vi "Full Stock venta.vi"(7 "Inventario/ventas":bool=TRUE, 8 "error in (no error)":errorcluster, 10 "Ubicacion":string, 11 "Full pedido":string[][](array[string])) -> (0 "error out":errorcluster, 3 "Sobrantes":string[][](array[string]))   [LabVIEW 2018]
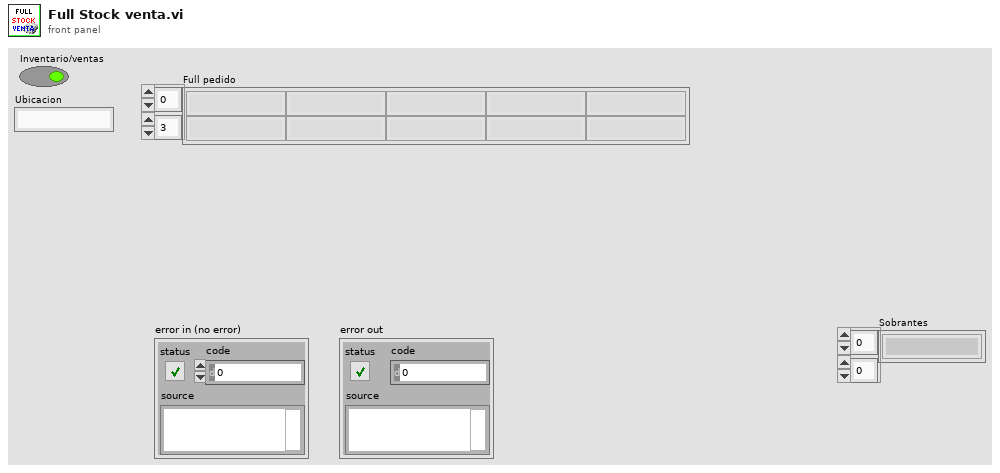
[diagram p1: front panel]
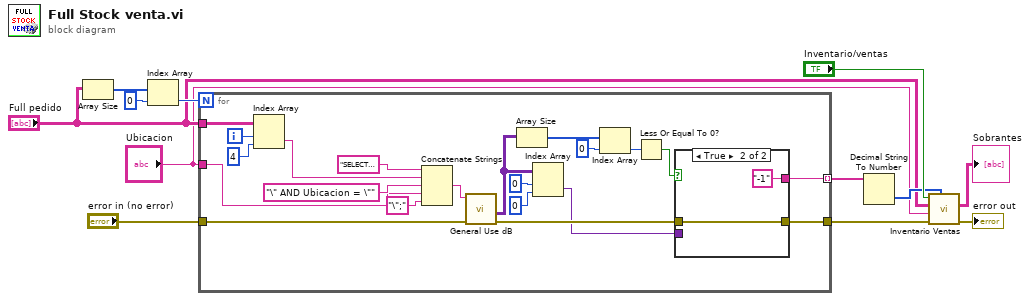
[diagram p0: block diagram]
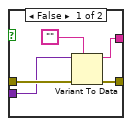
[diagram p2: hidden frame]
diagram:
  n1 = Array Size(array="Full pedido") -> (size(s)=w12:i32[])
  n2 = Index Array(array=w12, index=0) -> (element=w9:i32)
  n3 = for {
    N: w9 -> [_]
    tunnel: [w22] -> w4
    tunnel: "error in (no error)" -> [w24]
    tunnel: "Full pedido" -> [w32]
    tunnel: "Ubicacion" -> [w27]
    tunnel: [w18] -> w3 mode=indexing
    i -> [w30]
    n4 = Index Array(array=w32, index (row)=w30, index (col)=4 ("disabled index (col)")) -> (element=w29:string)
    n5 = Concatenate Strings("SELECT Cantidad FROM Inventario WHERE Codigo  = \"", w29, "\" AND Ubicacion = \"" ("string"), w27, "\";" ("string")) -> (w25:string)
    n6 = call "General Use dB.vi"("error in (no error)"=w24, "Query"=w25) -> ("error out"=w23:errorcluster, "Return Data"=w17:variant[][])  [unwired: 8 in]
    n7 = Array Size(array=w17) -> (size(s)=w16:i32[])
    n8 = Index Array(array=w17, index (row)=0, index (col)=0 ("disabled index (col)")) -> (element=w19:variant)
    n9 = Index Array(array=w16, index=0) -> (element=w14:i32)
    n10 = Less Or Equal To 0?(x=w14) -> (x <= 0?=w13:bool)
    n11 = case shown="True" w13 {
      tunnel: w23 -> [w38 w40]
      tunnel: [w37 w40] -> w22
      tunnel: w19 -> [w36 _]
      tunnel: [w34 "-1"] -> w18
      frame False {
        n12 = Variant To Data(error in=w38, type="", Variant=w36) -> (data=w34:string, error out=w37:errorcluster)
      }
      frame True {
      }
    }
  }
  n13 = Decimal String To Number(string=w3) -> (number=w7:i32[])  [unwired: 2 in, 1 out]
  n14 = call "Inventario Ventas.vi"("Array"=w7, "error in (no error)"=w4, "Ubicacion"="Ubicacion", "Full pedido"="Full pedido", "Inventario/ventas"="Inventario/ventas") -> ("error out"=→"error out":errorcluster, "Sobrantes"=→"Sobrantes":string[][])  [unwired: 5 in]
